vi "Nufern Digital Control Global.vi"() -> ()   [LabVIEW 2015]
uses:
  Nufern Digital Timing Control.ctl
panel:
  in  "Nufern Digital Timing Control":T1={"Fire"=FALSE, "Start A-Scan"=0, "Stop A-Scan"=0, "Reps per Fire"=1, "B-Scan Spacing"=1} {"B-Scan Spacing" min=0 max=5000; "Reps per Fire" min=1 max=5000}
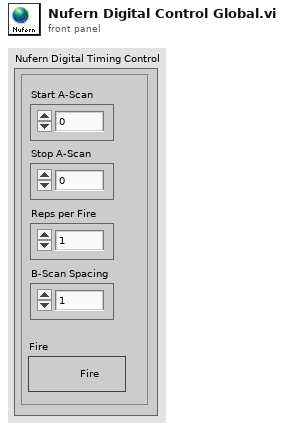
[diagram p1: front panel]
types:
  T1 = typedef "Nufern Digital Timing Control.ctl" = cluster{"Fire":bool, "Start A-Scan":u32, "Stop A-Scan":u32, "Reps per Fire":i32, "B-Scan Spacing":i32}
diagram:
